vi "Power Meter Check Status (No Objects).vi"(8 "error in (no error)":errorcluster, 10 "VISA resource name":refnum<visa-resource-name>, 11 "Cluster In":T2={"Wavelength"=0.0, "AVG"=0, "Range"=0, "Backlight"=0, "Beeper"=0, "Zero"=0, "Local Lockout"=0, "ATTN"=0, "Run/Stop"=0, "Units"=0, "Averaging Points"=0, "Averaging"=FALSE, "Most Recent Power"=5.5, "Filter"=1} {"AVG" items=["Slow"=1, "Medium"=2, "Fast"=3]; "Range" items=["Auto", "Lowest", "2", "3", "4", "5", "6", "7", "Highest"]; "Backlight" items=["Off", "Low", "High"]; "Beeper" items=["Off", "On"]; "Zero" items=["Off", "On"]; "Local Lockout" items=["Off", "On"]; "ATTN" items=["Off", "On"]; "Run/Stop" items=["Stop", "Run"]; "Units" items=["W"=1, "dB"=2, "dBm"=3, "REL"=4]; "Filter" items=["Orange"=1, "Green"=2, "Yellow"=3]}) -> (0 "error out":errorcluster, 1 "Status":string, 3 "Cluster Out":T2={"Wavelength"=0.0, "AVG"=0, "Range"=0, "Backlight"=0, "Beeper"=0, "Zero"=0, "Local Lockout"=0, "ATTN"=0, "Run/Stop"=0, "Units"=0, "Averaging Points"=0, "Averaging"=FALSE, "Most Recent Power"=5.5, "Filter"=1} {"AVG" items=["Slow"=1, "Medium"=2, "Fast"=3]; "Range" items=["Auto", "Lowest", "2", "3", "4", "5", "6", "7", "Highest"]; "Backlight" items=["Off", "Low", "High"]; "Beeper" items=["Off", "On"]; "Zero" items=["Off", "On"]; "Local Lockout" items=["Off", "On"]; "ATTN" items=["Off", "On"]; "Run/Stop" items=["Stop", "Run"]; "Units" items=["W"=1, "dB"=2, "dBm"=3, "REL"=4]; "Filter" items=["Orange"=1, "Green"=2, "Yellow"=3]})   [LabVIEW 2013]
doc: "(Dynamic) Check if the instrument is powered on and update its member fields with the instrument's current status. Optionally return a text status message."
uses:
  Public/Filters.ctl
  Newport 1830-C.lvlib
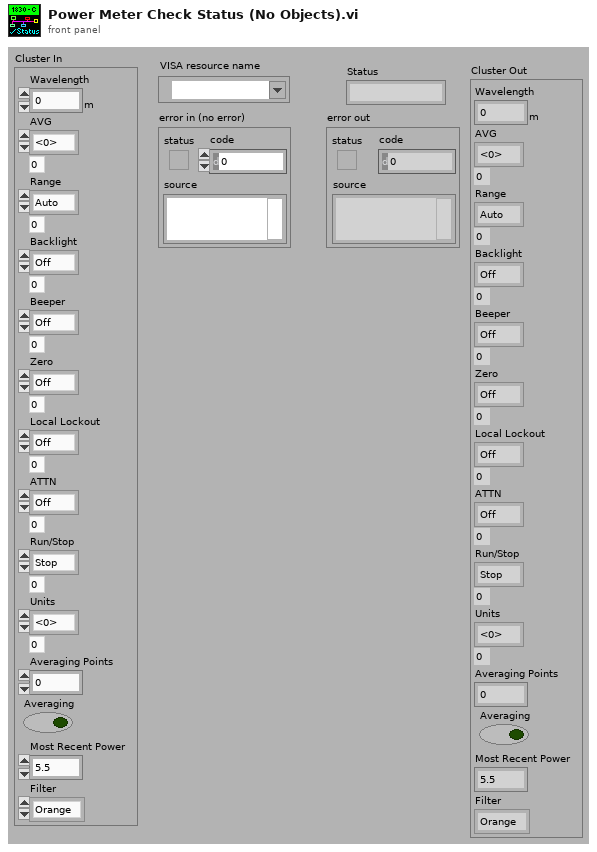
[diagram p1: front panel]
types:
  T1 = typedef "Newport 1830-C.lvlib/Filters.ctl" = u16
  T2 = cluster{"Wavelength":dbl[unit], "AVG":u16, "Range":u16, "Backlight":u16, "Beeper":u16, "Zero":u16, "Local Lockout":u16, "ATTN":u16, "Run/Stop":u16, "Units":u16, "Averaging Points":u32, "Averaging":bool, "Most Recent Power":dbl, "Filter":T1}
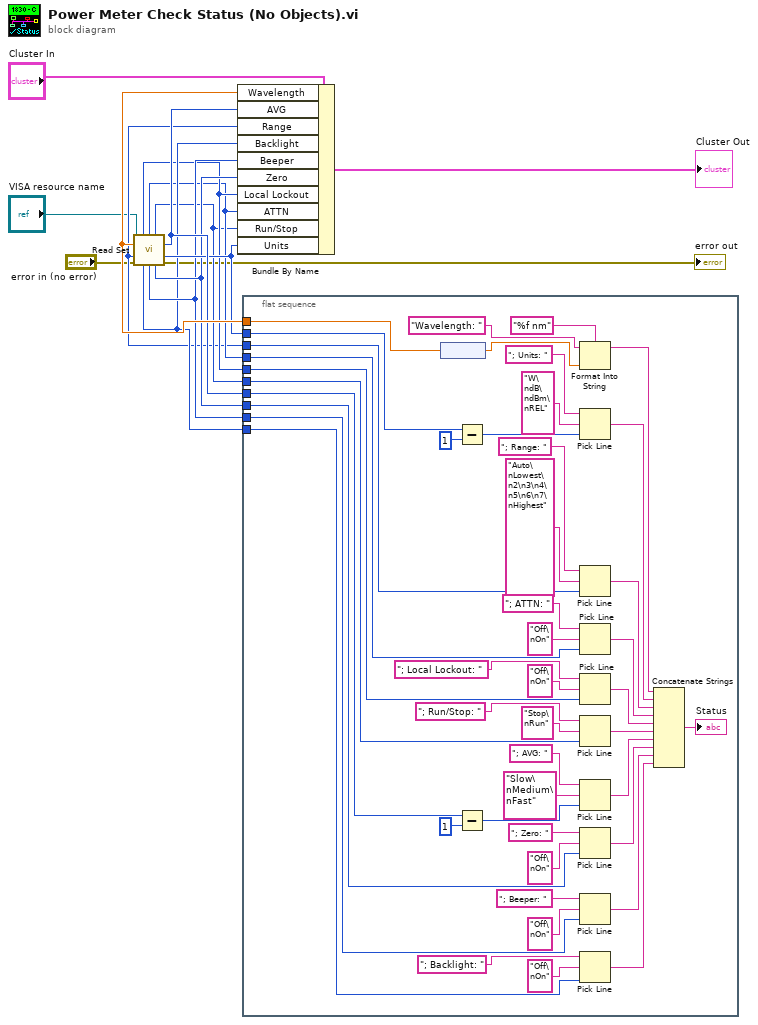
[diagram p0: block diagram]
diagram:
  n1 = call "Read Set.vi"("VISA resource name"="VISA resource name", "error in (no error)"="error in (no error)") -> ("Local Lockout"=w9:u32, "ATTN"=w8:u32, "Run/Stop"=w7:u32, "Wavelength (nnnn)"=w15:dbl[unit], "AVG"=w14:u32, "Range (1:8)"=w6:u32, "Units"=w13:u32, "Backlight"=w10:u32, "Beeper"=w11:u32, "Zero"=w12:u32, "error out"=→"error out":errorcluster)  [unwired: 2 in, 1 out]
  n2 = Bundle By Name(cluster="Cluster In", "Wavelength"=w15, "AVG"=w14, "Range"=w6, "Backlight"=w10, "Beeper"=w11, "Zero"=w12, "Local Lockout"=w9, "ATTN"=w8, "Run/Stop"=w7, "Units"=w13) -> (→"Cluster Out":T2)
  n3 = flat-sequence {
    tunnel: w13 -> [w53]
    tunnel: w15 -> [w49]
    tunnel: w8 -> [w47]
    tunnel: w6 -> [w43]
    tunnel: w9 -> [w39]
    tunnel: w7 -> [w35]
    tunnel: w14 -> [w31]
    tunnel: w12 -> [w25]
    tunnel: w11 -> [w21]
    tunnel: w10 -> [w17]
    frame #0 {
      n4 = node(w49) -> (w61:dbl)
      n5 = Subtract(x=w53, y=u32 1) -> (x-y=w51:u32)
      n6 = Subtract(x=w31, y=u32 1) -> (x-y=w29:u32)
      n7 = Format Into String(format string="%f nm", initial string="Wavelength: ", w61) -> (resulting string=w56:string)  [unwired: 1 in, 1 out]
      n8 = Pick Line(string ("")="; Units: ", multi-line string="W\ndB\ndBm\nREL", line index=w51) -> (output string=w55:string)
      n9 = Pick Line(string ("")="; Range: ", multi-line string="Auto\nLowest\n2\n3\n4\n5\n6\n7\nHighest", line index=w43) -> (output string=w42:string)
      n10 = Pick Line(string ("")="; ATTN: ", multi-line string="Off\nOn", line index=w47) -> (output string=w46:string)
      n11 = Pick Line(string ("")="; Local Lockout: ", multi-line string="Off\nOn", line index=w39) -> (output string=w38:string)
      n12 = Pick Line(string ("")="; Run/Stop: ", multi-line string="Stop\nRun", line index=w35) -> (output string=w34:string)
      n13 = Pick Line(string ("")="; AVG: ", multi-line string="Slow\nMedium\nFast", line index=w29) -> (output string=w28:string)
      n14 = Pick Line(string ("")="; Zero: ", multi-line string="Off\nOn", line index=w25) -> (output string=w24:string)
      n15 = Pick Line(string ("")="; Beeper: ", multi-line string="Off\nOn", line index=w21) -> (output string=w20:string)
      n16 = Pick Line(string ("")="; Backlight: ", multi-line string="Off\nOn", line index=w17) -> (output string=w16:string)
      n17 = Concatenate Strings(w56, w55, w42, w46, w38, w34, w28, w24, w20, w16) -> (→"Status":string)
    }
  }
